vi "Build_Asylum_ReadString.vi"(8 "error in (no error)":errorcluster, 11 "parameterName":string) -> (0 "error out":errorcluster, 3 "String":string)   [LabVIEW 2019]
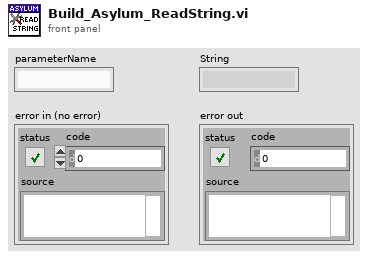
[diagram p1: front panel]
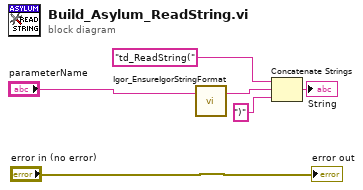
[diagram p0: block diagram]
diagram:
  n1 = call "Igor_EnsureIgorStringFormat.vi"("Value"="parameterName") -> ("Value"=w5:string)  [unwired: 2 in]
  n2 = Concatenate Strings("td_ReadString(" ("string"), w5, ")" ("string")) -> (→"String":string)
  "error out" <- "error in (no error)"
